vi "process_stim_NI.vi"(8 "error in (no error)":errorcluster) -> (0 "error out":errorcluster)   [LabVIEW 2010]
uses:
  typedefs/control_stim_enum.ctl
  typedefs/device_parameters.ctl
  typedefs/protocol_parameters.ctl
  <vilib>/DAQmx/write.llb/DAQmx Write (Analog 1D DBL 1Chan NSamp).vi
  <vilib>/daqmx/miscellaneous.llb/DAQmx Fill In Error Info.vi
  Program Files (x86)/National Instruments/LabVIEW 2010/resource/objmgr/daqmx.rc
panel:
  out "Waveform Graph":dbl[](graph)
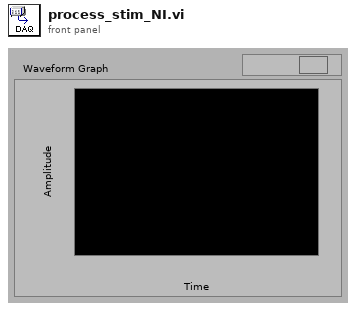
[diagram p1: front panel]
types:
  T1 = typedef "control_stim_enum.ctl" = enum16{"Init", "Stim", "Stop", "Quit"}
  T2 = cluster{"Control stim Enum":T1, "variant":variant}
  T3 = typedef "device_parameters.ctl" = cluster{"Triggered?":bool, "Shutter channel":tag, "Acquisition channels":tag, "Acquisition sample rate":dbl, "Pixels to integrate":i32, "Effective sample rate":dbl, "Read chunk size":i32, "Stimulation channel":tag, "Stimulation sample rate":dbl, "Write chunk size":i32}
  T4 = typedef "protocol_parameters.ctl" = cluster{"Repetitions":dbl, "ON time":dbl, "OFF time":dbl, "Stim onset":dbl, "Stim frequency":dbl, "Stim length":dbl, "Acquire before ON":dbl, "Acquire after ON":dbl, "Sync shutter to acquisition":bool}
  T5 = cluster{"Device parameters":T3, "Protocol parameters":T4}
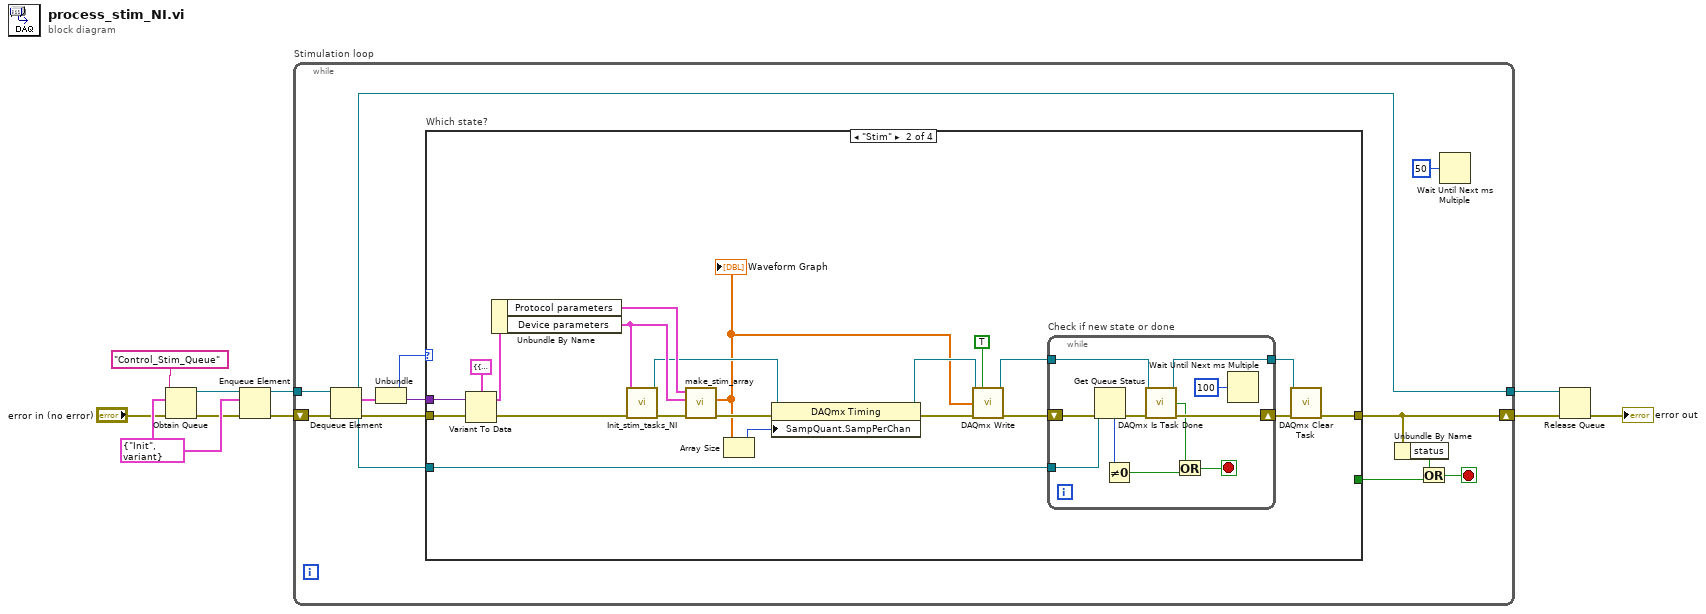
[diagram p0: block diagram]
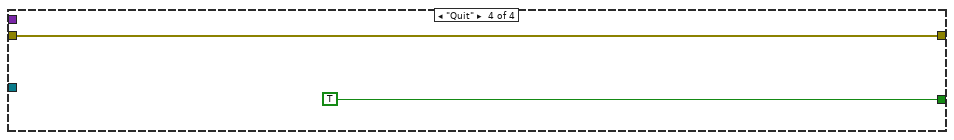
[diagram p4: hidden frame]
diagram:
  w10 = T2 {"Control stim Enum"=enum."Init", "variant"=variant} ("ControlDAQ state cluster")
  n1 = Obtain Queue(name (unnamed)="Control_Stim_Queue", element data type=w10, error in (no error)="error in (no error)") -> (queue out=w6:refnum<queue>, error out=w8:errorcluster)  [unwired: 2 in, 1 out]
  n2 = Enqueue Element(queue=w6, element=w10, error in (no error)=w8) -> (queue out=w7:refnum<queue>, error out=w9:errorcluster)  [unwired: 1 in, 1 out]
  n3 = while "Stimulation loop" {
    shift-right: [w16] -> w5
    shift-left: w9 -> [w21]
    tunnel: w7 -> [w22]
    tunnel: [w11] -> w4
    stop <- w14 stop-if-true
    n4 = Dequeue Element(queue=w22, error in (no error)=w21) -> (queue out=w11:refnum<queue>, element=w20:T2, error out=w18:errorcluster)  [unwired: 1 in, 1 out]
    n5 = Unbundle(w20) -> ("Control stim Enum"=w13:T1, "variant"=w19:variant)
    n6 = case "Which state?" shown="\"Stim\"" w13 {
      tunnel: w11 -> [_ w41 _ _]
      tunnel: w19 -> [_ w44 _ _]
      tunnel: w18 -> [w23 w43 w56 w57]
      tunnel: [w23 w42 w56 w57] -> w16
      tunnel: [_ _ _ TRUE] -> w17
      frame "Init", Default {
      }
      frame "Stim" {
        n7 = Variant To Data(error in=w43, Variant=w44, type=T5 {"Device parameters"={"Triggered?"=FALSE, "Shutter channel"="", "Acquisition channels"="", "Acquisition sample rate"=100.0, "Pixels to integrate"=0, "Effective sample rate"=100.0, "Read chunk size"=0, "Stimulation channel"="", "Stimulation sample rate"=100.0, "Write chunk size"=0}, "Protocol parameters"={"Repetitions"=1.0, "ON time"=40.0, "OFF time"=120.0, "Stim onset"=5.0, "Stim frequency"=1.0, "Stim length"=1.0, "Acquire before ON"=1.0, "Acquire after ON"=0.0, "Sync shutter to acquisition"=FALSE}}) -> (error out=w40:errorcluster, data=w37:T5)
        n8 = Unbundle By Name(w37) -> ("Protocol parameters"=w36:T4, "Device parameters"=w35:T3)
        n9 = call "Init_stim_tasks_NI.vi"("error in"=w40, "Device parameters"=w35) -> ("error out"=w39:errorcluster, "Stim task out"=w33:refnum<k21>)  [unwired: 6 in]
        n10 = call "make_stim_array.vi"("Error in"=w39, "Device parameters"=w35, "Protocol parameters"=w36) -> ("Error out"=w34:errorcluster, "Stim array"=w31:dbl[])  [unwired: 7 in]
        "Waveform Graph" <- w31
        n11 = Array Size(array=w31) -> (size(s)=w30:i32)
        n12 = property class="DAQmx Timing"(reference=w33, error in=w34, "SampQuant.SampPerChan"=w30) -> (reference out=w32:refnum<k21>, error out=w28:errorcluster)
        n13 = call-poly <vilib>:"DAQmx Write.vi"("task/channels in"=w32, "auto start"=TRUE, "data"=w31, "error in"=w28) -> ("task out"=w26:refnum<k21>, "error out"=w27:errorcluster)  [unwired: 9 in, 1 out]
        n14 = while "Check if new state or done" {
          tunnel: w41 -> [w55]
          tunnel: w26 -> [w51]
          tunnel: [w50] -> w25
          shift-right: [w52] -> w24
          shift-left: w27 -> [w54]
          stop <- w46 stop-if-true
          n15 = Get Queue Status(queue=w55, error in (no error)=w54) -> (error out=w53:errorcluster, # elements in queue=w49:i32)  [unwired: 1 in, 6 out]
          n16 = Not Equal To 0?(x=w49) -> (x != 0?=w47:bool)
          n17 = call <vilib>:"DAQmx Is Task Done.vi"("task/channels in"=w51, "error in"=w53) -> ("task out"=w50:refnum<k21>, "task done?"=w48:bool, "error out"=w52:errorcluster)  [unwired: 11 in]
          n18 = Or(x=w48, y=w47) -> (x .or. y?=w46:bool)
          n19 = Wait Until Next ms Multiple(millisecond multiple=u32 100) -> ()  [unwired: 1 out]
        }
        n20 = call <vilib>:"DAQmx Clear Task.vi"("task in"=w25, "error in"=w24) -> ("error out"=w42:errorcluster)  [unwired: 13 in]
      }
      frame "Stop" {
      }
      frame "Quit" {
      }
    }
    n21 = Unbundle By Name(w16) -> ("status"=w15:bool)
    n22 = Or(x=w15, y=w17) -> (x .or. y?=w14:bool)
    n23 = Wait Until Next ms Multiple(millisecond multiple=u32 50) -> ()  [unwired: 1 out]
  }
  n24 = Release Queue(queue=w4, error in (no error)=w5) -> (error out=→"error out":errorcluster)  [unwired: 1 in, 2 out]
